vi "SigProc_subVI getBinRange.vi"(1 "Y Data":dbl[](array[numeric])) -> (0 "Valid Data":dbl[](array[numeric]))   [LabVIEW 2018, in "Sig2MS.lvclass"]
uses:
  Sig2MS.lvclass
  <vilib>/Analysis/NI_AALBase.lvlib
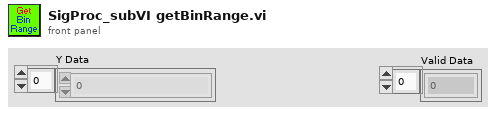
[diagram p1: front panel]
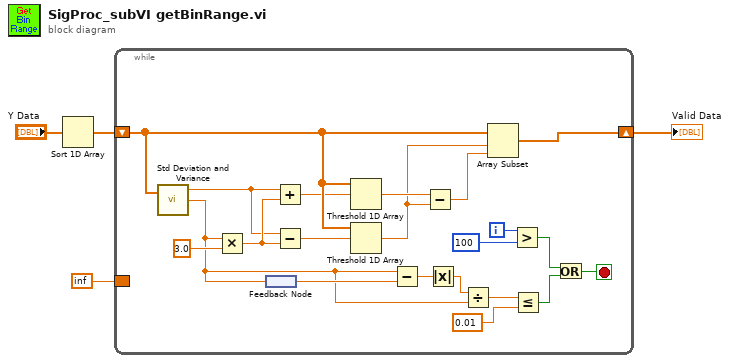
[diagram p0: block diagram]
diagram:
  n1 = Sort 1D Array(array="Y Data") -> (sorted array=w3:dbl[])
  n2 = while {
    shift-right: [w20] -> w1
    shift-left: w3 -> [w21]
    border: inf ("standard deviation") -> [_]
    i -> [w12]
    stop <- w13 stop-if-true
    n3 = call <vilib>:"Std Deviation and Variance.vi"("X"=w21) -> ("mean"=w7:dbl, "standard deviation"=w16:dbl)  [unwired: 1 in, 1 out]
    n4 = Multiply(x=w16, y=3.0) -> (x*y=w8:dbl)
    n5 = feedback-in #1(w16) -> ()
    n6 = feedback #1() -> (w19:dbl)
    n7 = Add(x=w7, y=w8) -> (x+y=w9:dbl)
    n8 = Subtract(x=w7, y=w8) -> (x-y=w10:dbl)
    n9 = Threshold 1D Array(2:w9, 3:w21) -> (0:w24:dbl)  [unwired: 1 in]
    n10 = Threshold 1D Array(2:w10, 3:w21) -> (0:w23:dbl)  [unwired: 1 in]
    n11 = Subtract(x=w16, y=w19) -> (x-y=w18:dbl)
    n12 = Subtract(x=w24, y=w23) -> (x-y=w22:dbl)
    n13 = Absolute Value(x=w18) -> (abs(x)=w17:dbl)
    n14 = Divide(x=w17, y=w16) -> (x/y=w15:dbl)
    n15 = Array Subset(array=w21, index=w23, length=w22) -> (w20:dbl[])
    n16 = Greater?(x=w12, y=100) -> (0:w6:bool)
    n17 = Less Or Equal?(x=w15, y=0.01) -> (x <= y?=w5:bool)
    n18 = Or(x=w6, y=w5) -> (x .or. y?=w13:bool)
  }
  "Valid Data" <- w1
